vi "Constants_Globals.vi"() -> ()   [LabVIEW 2019]
panel:
  in  "Robot_Length(in)":dbl=28.0
  in  "Robot_Width(in)":dbl=28.0
  in  "Max_Ground_Speed (ft/s)":dbl=14.0
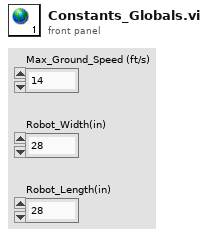
[diagram p1: front panel]
diagram:
